vi "Core.vi"(8 "error in":errorcluster, 9 "Structure Type":T1, 10 "T: Replace / F: Enclose":bool, 11 "VI in":refnum<vi>) -> (0 "error out":errorcluster, 3 "VI out":refnum<vi>)   [LabVIEW 2020, in "Enclose in Structure.lvlib"]
uses:
  Enclose in Structure.lvlib
  Structure Type.ctl
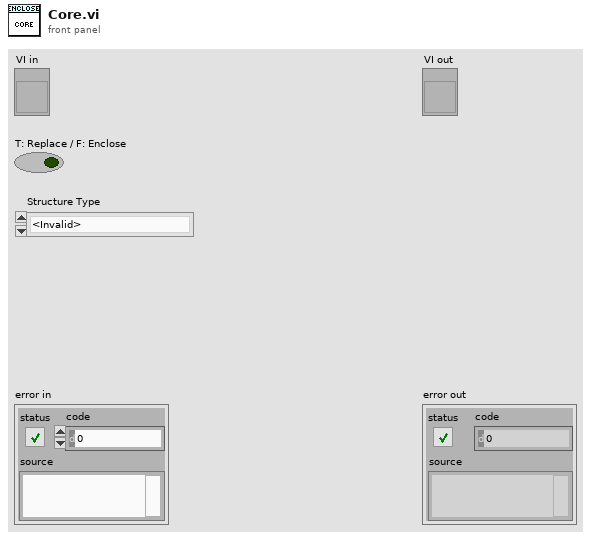
[diagram p1: front panel]
types:
  T1 = typedef "Enclose in Structure.lvlib/Structure Type.ctl" = enum16{"<Invalid>", "For Loop", "While Loop", "Timed Loop", "Timed Sequence", "Case Structure", "Event Structure", "In Place Element Structure", "Flat Sequence", "Diagram Disable Structure", "Conditional Disable Structure", "Type Specialization Structure"}
  T2 = typedef "LVRectTypeDef.ctl" = cluster{"Left":i16, "Top":i16, "Right":i16, "Bottom":i16}
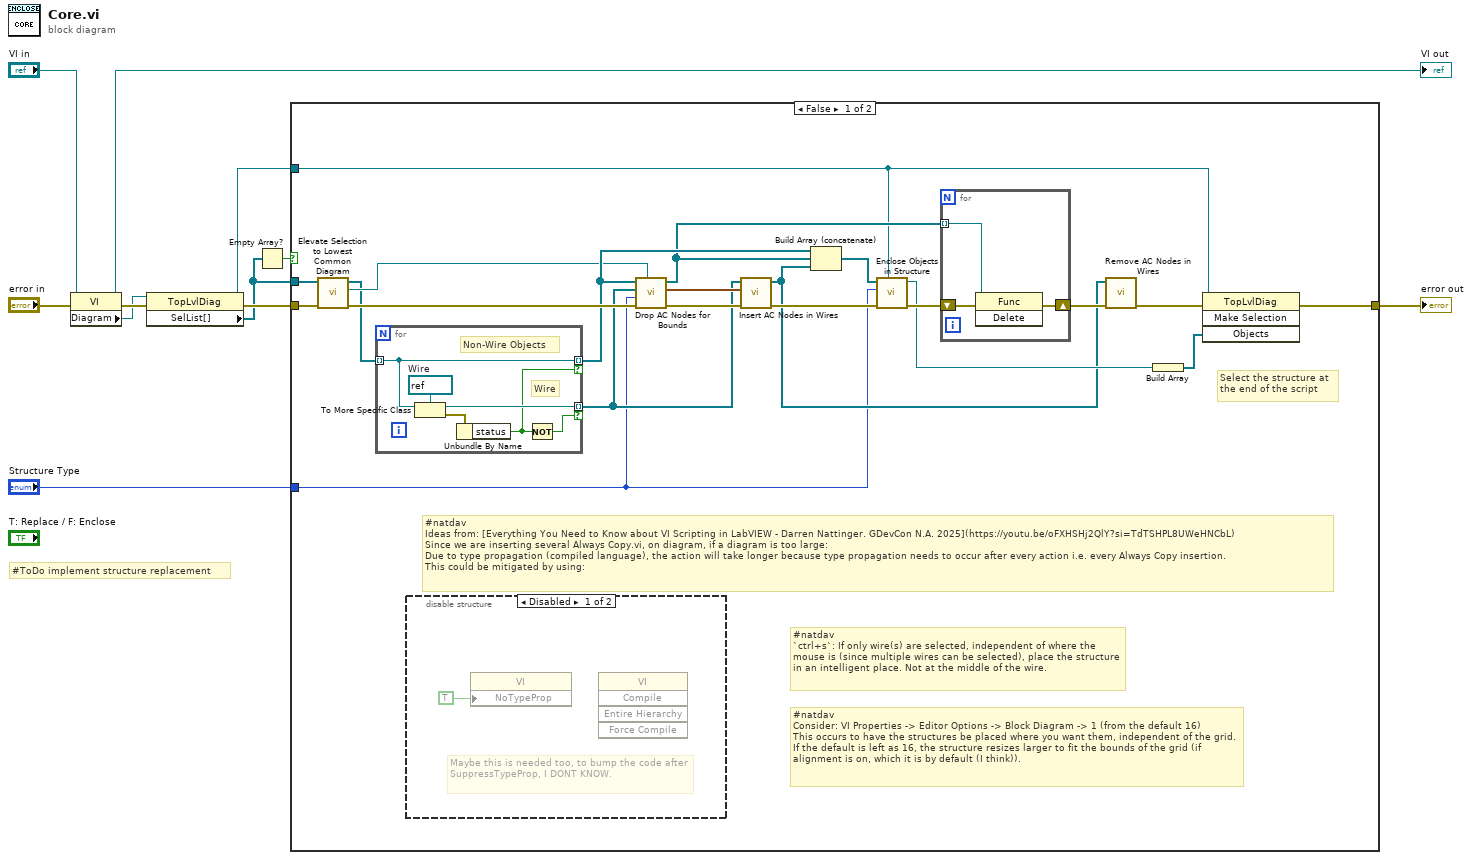
[diagram p0: block diagram]
diagram:
  # "#ToDo implement structure replacement"
  n1 = property class="VI"(reference="VI in", error in="error in") -> (reference out=→"VI out":refnum<vi>, error out=w10:errorcluster, "Diagram"=w9:refnum<vi>)
  n2 = property class="TopLvlDiag"(reference=w9, error in=w10) -> (reference out=w3:refnum<vi>, error out=w4:errorcluster, "SelList[]"=w2:refnum<vi>[])
  n3 = Empty Array?(array=w2) -> (empty?=w1:bool)
  n4 = case shown="False" w1 {
    tunnel: [w22 w43] -> w6
    tunnel: "Structure Type" -> [w18 _]
    tunnel: w4 -> [w17 w43]
    tunnel: w3 -> [w16 _]
    tunnel: w2 -> [w13 _]
    frame False {
      # "#natdav\n`ctrl+s`: If only wire(s) are selected, independent of where the mouse is (since multiple wires can be selected), place the structure in an intelligent place. Not at the middle of the wire."
      # "#natdav\nConsider: VI Properties -> Editor Options -> Block Diagram -> 1 (from the default 16)\nThis occurs to have the structures be placed where you want them, independent of the grid. If the default is left as 16, the structure resizes larger to fit the bounds of the grid (if alignment is on, which it is by default (I think))."
      # "#natdav\nIdeas from: [Everything You Need to Know about VI Scripting in LabVIEW - Darren Nattinger. GDevCon N.A. 2025](https://youtu.be/oFXHSHj2QlY?si=TdTSHPL8UWeHNCbL)\nSince we are inserting several Always Copy.vi, on diagram, if a diagram is too large:\nDue to type propagation (compiled language), the action will take longer because type propagation needs to occur after every action i.e. every Always Copy insertion.\nThis could be mitigated by using:"
      # "Select the structure at the end of the script"
      n5 = call "Elevate Selection to Lowest Common Diagram.vi"("error in"=w17, "Selection in"=w13) -> ("error out"=w31:errorcluster, "Lowest Common Diagram"=w15:refnum<vi>, "Selection out"=w12:refnum<vi>[])  [unwired: 7 in]
      n6 = for {
        tunnel: [w37] -> w26 mode=indexing if=w35
        tunnel: [w34] -> w25 mode=indexing if=w36
        tunnel: w12 -> [w34] mode=indexing
        w39 = refnum<vi> refnum  # Wire
        # "Wire"
        # "Non-Wire Objects"
        n7 = To More Specific Class(target class=w39, reference=w34) -> (specific class reference=w37:refnum<vi>, error out=w38:errorcluster)  [unwired: 1 in]
        n8 = Unbundle By Name(w38) -> ("status"=w36:bool)
        n9 = Not(x=w36) -> (.not. x?=w35:bool)
      }
      n10 = disable-structure shown="Disabled" {
        frame Disabled {
          # "Maybe this is needed too, to bump the code after SuppressTypeProp, I DONT KNOW."
          n11 = property class="VI"("NoTypeProp"=TRUE ("Suppress Type Prop")) -> ()  [unwired: 2 in, 2 out]
          n12 = invoke class="VI" method="Compile"() -> ()  [unwired: 5 in, 5 out]
        }
        frame Enabled {
        }
      }
      n13 = call "Drop AC Nodes for Bounds.vi"("Diagram"=w15, "error in"=w31, "Structure Type"=w18, "Wires"=w26, "Non-Wire Objects"=w25) -> ("error out"=w29:errorcluster, "Bounds"=w27:T2, "Always Copy Nodes"=w24:refnum<vi>[])  [unwired: 4 in]
      n14 = call "Insert AC Nodes in Wires.vi"("error in"=w29, "Bounds"=w27, "Wires"=w26) -> ("error out"=w32:errorcluster, "Always Copy Nodes"=w19:refnum<vi>[])  [unwired: 7 in]
      n15 = Build Array (concatenate)(w25, w24, w19) -> (w14:refnum<vi>[])
      n16 = call "Enclose Objects in Structure.vi"("Top Level Diagram"=w16, "error in"=w32, "Structure Type"=w18, "Objects"=w14) -> ("error out"=w28:errorcluster, "Structure"=w20:refnum<vi>)  [unwired: 6 in]
      n17 = for {
        shift-right: [w41] -> w30
        shift-left: w28 -> [w42]
        tunnel: w24 -> [w40] mode=indexing
        n18 = invoke class="Func" method="Delete"(reference=w40, error in=w42) -> (error out=w41:errorcluster)  [unwired: 1 in, 2 out]
      }
      n19 = call "Remove AC Nodes in Wires.vi"("error in"=w30, "Always Copy Nodes"=w19) -> ("error out"=w23:errorcluster)  [unwired: 9 in]
      n20 = Build Array(w20) -> (w21:refnum<vi>[])
      n21 = invoke class="TopLvlDiag" method="Make Selection"(reference=w16, error in=w23, "Objects"=w21) -> (error out=w22:errorcluster)  [unwired: 1 in, 3 out]
    }
    frame True {
    }
  }
  "error out" <- w6
